vi "Save Settings AH2700A (SubVI).vi"(8 "error in (no error)":errorcluster, 11 "Instrument parameters (in)":T1) -> (0 "error out":errorcluster, 2 "appended array":string[][](array[string]), 3 "VISA Refnum out":refnum<visa-resource-name>)   [LabVIEW 2025]
uses:
  TYPE DEFS/S2DS_Instrument parameters.ctl
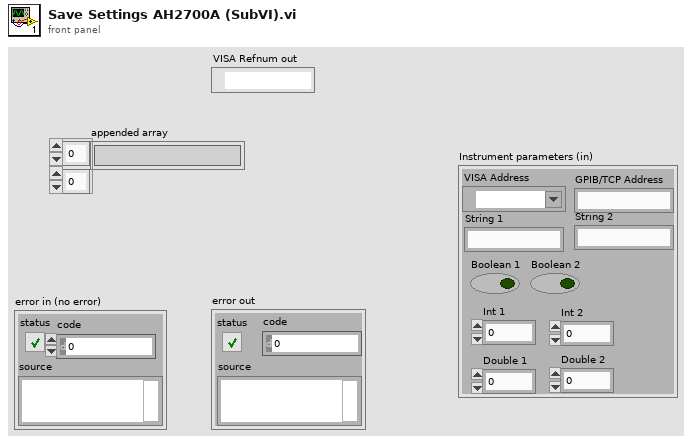
[diagram p1: front panel]
types:
  T1 = typedef "S2DS_Instrument parameters.ctl" = cluster{"VISA Address":refnum<visa-resource-name>, "GPIB/TCP Address":string, "String 1":string, "String 2":string, "Boolean 1":bool, "Boolean 2":bool, "Int 1":i32, "Int 2":i32, "Double 1":dbl, "Double 2":dbl}
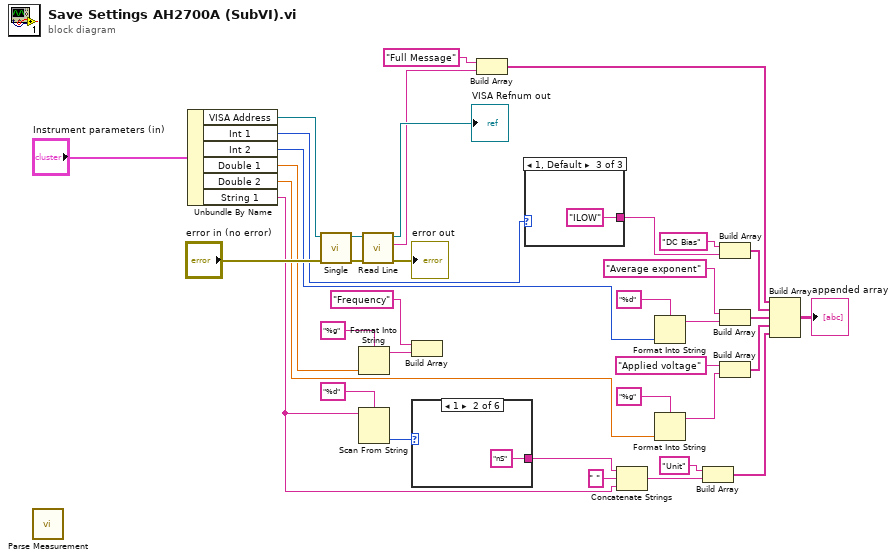
[diagram p0: block diagram]
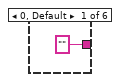
[diagram p2: hidden frame]
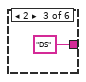
[diagram p3: hidden frame]
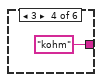
[diagram p4: hidden frame]
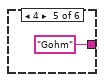
[diagram p5: hidden frame]
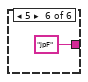
[diagram p6: hidden frame]
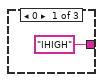
[diagram p7: hidden frame]
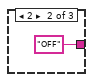
[diagram p8: hidden frame]
diagram:
  n1 = call "Parse Measurement.vi"() -> ()  [unwired: 11 in, 9 out]
  n2 = Unbundle By Name("Instrument parameters (in)") -> ("VISA Address"=w27:refnum<visa-resource-name>, "Int 1"=w23:i32, "Int 2"=w20:i32, "Double 1"=w16:dbl, "Double 2"=w13:dbl, "String 1"=w3:string)
  n3 = call "Single.vi"("error in"="error in (no error)", "VISA resource name"=w27) -> ("error out"=w35:errorcluster, "VISA resource name out"=w34:refnum<visa-resource-name>)  [unwired: 8 in]
  n4 = Format Into String(format string="%g", w16) -> (resulting string=w14:string)  [unwired: 2 in, 1 out]
  n5 = Scan From String(format string="%d", input string=w3) -> (output 1=w6:i32)  [unwired: 3 in, 3 out]
  n6 = call "Read Line.vi"("error in"=w35, "VISA resource name"=w34) -> ("error out"=→"error out":errorcluster, "Message"=w31:string, "VISA resource name out"=→"VISA Refnum out":refnum<visa-resource-name>)  [unwired: 5 in, 2 out]
  n7 = Build Array("Frequency", w14) -> ()  [unwired: 1 out]
  n8 = case shown="1" w6 {
    tunnel: ["" "nS" "DS" "kohm" "Gohm" "jpF"] -> w5
    frame 0, Default {
    }
    frame 1 {
    }
    frame 2 {
    }
    frame 3 {
    }
    frame 4 {
    }
    frame 5 {
    }
  }
  n9 = Build Array("Full Message", w31) -> (w30:string[])
  n10 = case shown="1, Default" w23 {
    tunnel: ["IHIGH" "OFF" "ILOW"] -> w22
    frame 0 {
    }
    frame 2 {
    }
    frame 1, Default {
    }
  }
  n11 = Concatenate Strings(w5, " " ("string"), w3) -> (w2:string)
  n12 = Format Into String(format string="%d", w20) -> (resulting string=w19:string)  [unwired: 2 in, 1 out]
  n13 = Format Into String(format string="%g", w13) -> (resulting string=w11:string)  [unwired: 2 in, 1 out]
  n14 = Build Array("Unit" ("element"), w2) -> (w1:string[])
  n15 = Build Array("DC Bias", w22) -> (w26:string[])
  n16 = Build Array("Average exponent", w19) -> (w18:string[])
  n17 = Build Array("Applied voltage" ("element"), w11) -> (w9:string[])
  n18 = Build Array(w30, w26, w18, w9, w1) -> (→"appended array":string[][])
